vi "Initialize Front Panel.vi"(8 "error in (no error)":errorcluster, 11 "IViewable in":refnum<class "IViewable.lvclass">) -> (0 "error out":errorcluster, 3 "IViewable out":refnum<class "IViewable.lvclass">)   [LabVIEW 2015, in "IViewable.lvlib" / "IViewable.lvclass"]
doc: "<License>\nCopyright © 2017 Composed Systems, LLC | All rights reserved\nwww.composed.io\n\nAuthor: Ethan Stern <ethan.stern@composed.io>\n\nThis software is provided \"AS IS\" WITHOUT WARRANTIES, either express or implied, AND IS FOR EDUCATIONAL PURPOSES ONLY.\n</License>"
uses:
  IViewable.lvclass
  IViewable.lvclass/IViewable.ctl
  ApplicationStyleReference/ApplicationStyleReference.lvclass/ApplicationStyleReference.ctl
  IApplicationStyle/IApplicationStyle.lvclass
  ApplicationStyleReference/ApplicationStyleReference.lvclass
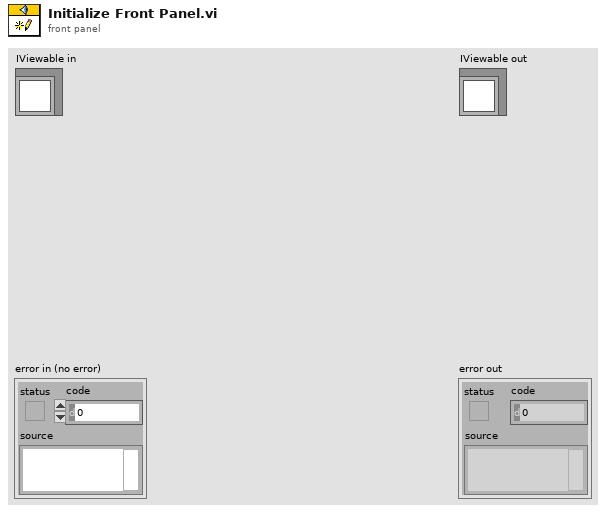
[diagram p1: front panel]
types:
  T1 = typedef "IViewable.lvlib/ApplicationStyleReference.lvclass/Application Style Reference.ctl" = refnum<data-value>
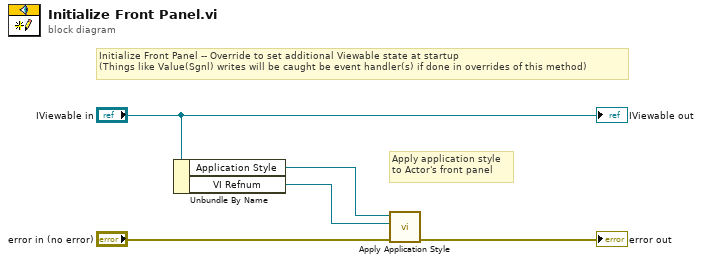
[diagram p0: block diagram]
diagram:
  # "Apply application style\nto Actor's front panel"
  # "Initialize Front Panel -- Override to set additional Viewable state at startup\n(Things like Value(Sgnl) writes will be caught be event handler(s) if done in overrides of this method)"
  n1 = Unbundle By Name("IViewable in") -> ("Application Style"=w2:T1, "VI Refnum"=w1:refnum<vi>)
  n2 = call "Apply Application Style.vi"("error in (no error)"="error in (no error)", "VI Refnum"=w1, "ApplicationStyleReference in"=w2) -> ("error out"=→"error out":errorcluster)  [unwired: 8 in]
  "IViewable out" <- "IViewable in"
